vi "Measurement UI.vi"() -> ()   [LabVIEW 2021, in "Line Transient Response with Pin Map UI.lvlib"]
uses:
  Line Transient Response with Pin Map UI.lvlib
  <instrlib>/niScope/Controls/niScope vertical coupling.ctl
  common/UI/controls/UI Scope Parameters.ctl
  common/PMIC Common.lvlib
panel:
  in  "MeasGraphs":T1(tab)
  out "MeasTable":string[][](table)
  out "InputVoltageV/STimeGraph":waveform(dbl)(graph) caption="Load Transient"
  out "OutputVoltageV/STimeGraph":waveform(dbl)(graph) caption="Load Transient"
  in  "Source Voltage v/s Time":string="SOURCE VOLTAGE vs TIME"
  in  "Output Voltage v/s Time":string="LOAD VOLTAGE vs TIME"
  out "ScopeGraph":T2(graph)
  out "waveform pins":string[](array[string])
  in  "enforce realtime":bool[](array[boolean])
  in  "reference position":dbl[](array[numeric]) caption="MIN SAMPLE RATE"
  in  "channel enabled":bool[](array[boolean])
  out "waveform length array":i32[](array[numeric])
  out "waveform dt array":dbl[](array[numeric])
  out "concatenated waveform Y":dbl[](array[numeric])
  out "waveform t0 array":dbl[](array[numeric])
  out "waveform sites":i32[](array[numeric])
  in  "vertical range":dbl[](array[numeric]) caption="VERTICAL RANGE"
  in  "vertical offset":dbl[](array[numeric]) caption="VERTICAL OFFSET"
  in  "probe attenuation":dbl[](array[numeric]) caption="PROBE ATTENUATION"
  in  "vertical coupling":T3[](array[typedef]) caption="VERTICAL COUPLING" items=["AC", "DC", "Ground"]
  in  "input impedance":u32[](array[ring]) caption="INPUT IMPEDANCE" items=["1 mega ohm"=0, "50 ohms"=2]
  in  "max input frequency":dbl[](array[numeric]) caption="MAX INPUT FREQUENCY"
  in  "min sample rate":dbl[](array[numeric]) caption="MIN SAMPLE RATE"
  in  "min record length":i32[](array[numeric]) caption="MIN RECORD LENGTH"
  in  "Pin Names for Scope":string[](array[string]) caption="PIN NAMES"
  out "Overshoot load voltage":dbl
  out "Undershoot load voltage":dbl
  out "Scope amplitudes":dbl[](array[numeric])
  in  "Load transient response":i32(ring)=1042 items=["Slow"=1041, "Normal"=1038, "Fast"=1039, "Custom"=1042]
  out "dt":dbl
  out "Load voltages":dbl[](array[numeric])
  out "Source voltages":dbl[](array[numeric])
  in  "Source transient response":i32(ring)=1042 items=["Slow"=1041, "Normal"=1038, "Fast"=1039, "Custom"=1042]
  in  "Open Scope Dialog":bool
  in  "Load pin name":string caption="LOAD PIN NAME"
  in  "Source pin name":string caption="SOURCE PIN NAME"
  in  "Source model":enum16{"NI PXIe-4151", "NI PXIe-4139"}(ring) caption="RESOURCE MODEL"
  in  "Scope configuration":string="Scope configuration"
  in  "Source voltage delay t2":dbl=0.005 caption="DELAY T2" format="%#_6ps"
  in  "Source voltage delay t1":dbl=0.005 caption="DELAY T1" format="%#_6ps"
  in  "Source voltatge pulse duration":dbl=0.005 caption="PULSE DURATION" format="%#_6ps"
  in  "Source voltage rising slew rate":dbl=50000.0 caption="VOLTAGE RISING SLEW RATE" format="%#_6pV/s"
  in  "Source voltage falling slew rate":dbl=50000.0 caption="VOLTAGE FALLING SLEW RATE" format="%#_6pV/s"
  in  "Source maximum power":dbl=300.0 caption="MAXIMUM POWER" format="%#_6pW"
  in  "Source current limit":dbl=0.25 caption="CURRENT LIMIT" format="%#_6pA"
  in  "Load configuration":string="Load configuration"
  in  "Source configuration":string="Source configuration"
  in  "Source voltage set point 2":dbl=20.0 caption="VOLTAGE SET POINT 2" format="%#_6pV"
  in  "Source voltage set point 1":dbl=7.0 caption="VOLTAGE SET POINT 1" format="%#_6pV"
  in  "Source voltage pole-zero ratio":dbl=2.0 caption="POLE-ZERO RATIO"
  in  "Source voltage gain bandwidth":dbl=2000.0 caption="GAIN BANDWIDTH" format="%#_6pHz"
  in  "Source voltage compensation frequency":dbl=3530.0 caption="COMP. FREQUENCY" format="%#_6pHz"
  in  "Source fast":bool
  in  "Source normal":bool
  in  "Source slow":bool
  in  "Source SourceAdapt":string="Voltage SourceAdapt Parameters"
  in  "Load voltage limit range":dbl=4.0 caption="VOLTAGE LIMIT RANGE" format="%#_6pV"
  in  "Load current level range":dbl=4.0 caption="CURRENT LEVEL RANGE" format="%#_6pA"
  in  "Load current pole-zero ratio":dbl=0.3 caption="POLE-ZERO RATIO"
  in  "Load current gain bandwidth":dbl=14000.0 caption="GAIN BANDWIDTH" format="%#_6pHz"
  in  "Load current compensation frequency":dbl=180000.0 caption="COMP. FREQUENCY" format="%#_6pHz"
  in  "Source sample rate":dbl=1800000.0 caption="SAMPLE RATE" format="%#_6pS/s"
  in  "Load current level":dbl=0.03 caption="CURRENT LEVEL" format="%#_6pA"
  in  "Load fast":bool
  in  "Load normal":bool
  in  "Load slow":bool
  in  "Load SourceAdapt":string="Current SourceAdapt Parameters"
  in  "DUT setup time":dbl=1.0 caption="DUT SETUP TIME" format="%#_6ps"
  in  "Measurement settings":string="Measurement settings"
  in  "Nominal output voltage":dbl=3.3 caption="NOMINAL O/P VOLTAGE" format="%#_6pV"
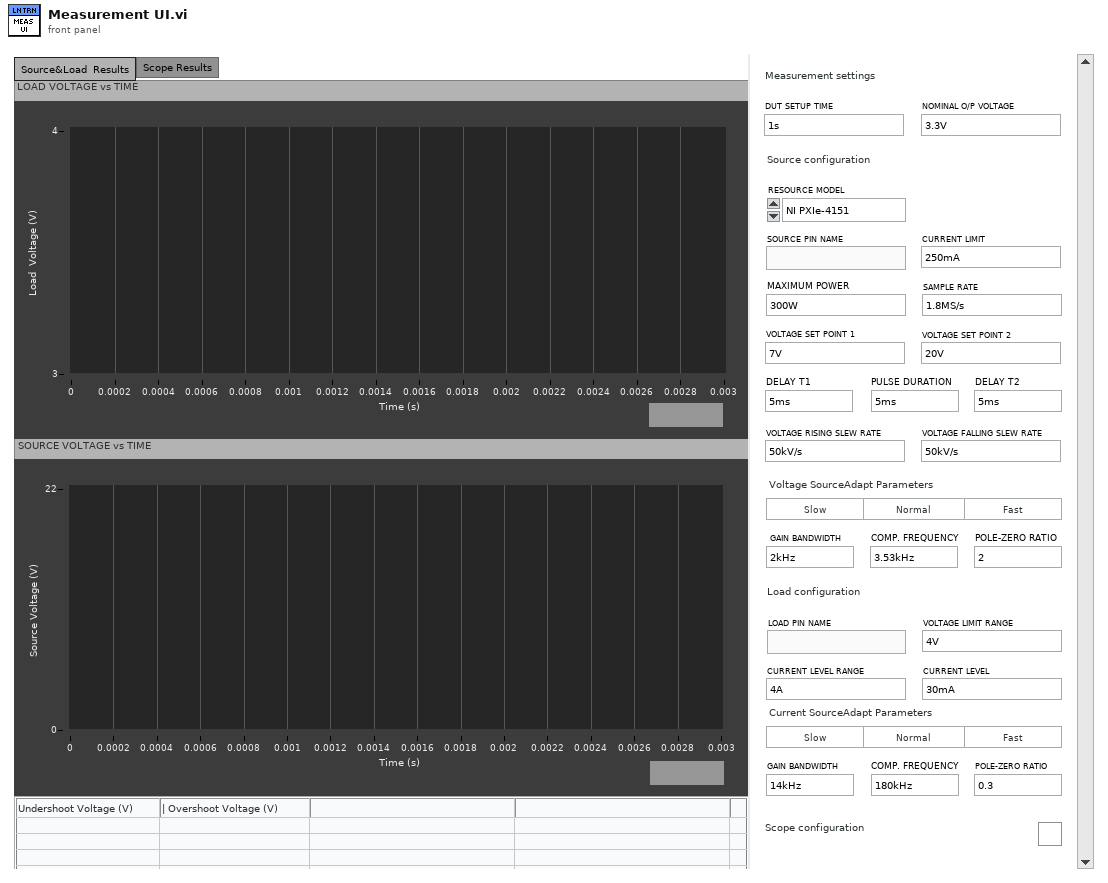
[diagram p1: front panel]
types:
  T1 = enum32{"Source&Load  Results", "Scope Results", "Hidden Controls"}
  T2 = cluster{"Load currents":dbl[], "Efficiency":dbl[]}[]
  T3 = typedef "niScope vertical coupling.ctl" = i32
  T4 = typedef "PMIC Common.lvlib/UI Scope Parameters.ctl" = cluster{"Pin name":string, "Vertical range":dbl, "Vertical offset":dbl, "Probe attenuation":dbl, "Vertical coupling":i32, "Channel enabled":bool, "Input impedance":u32, "Max input frequency":dbl, "Min sample rate":dbl, "Reference position":dbl, "Min record length":i32, "Enforce realtime":bool}
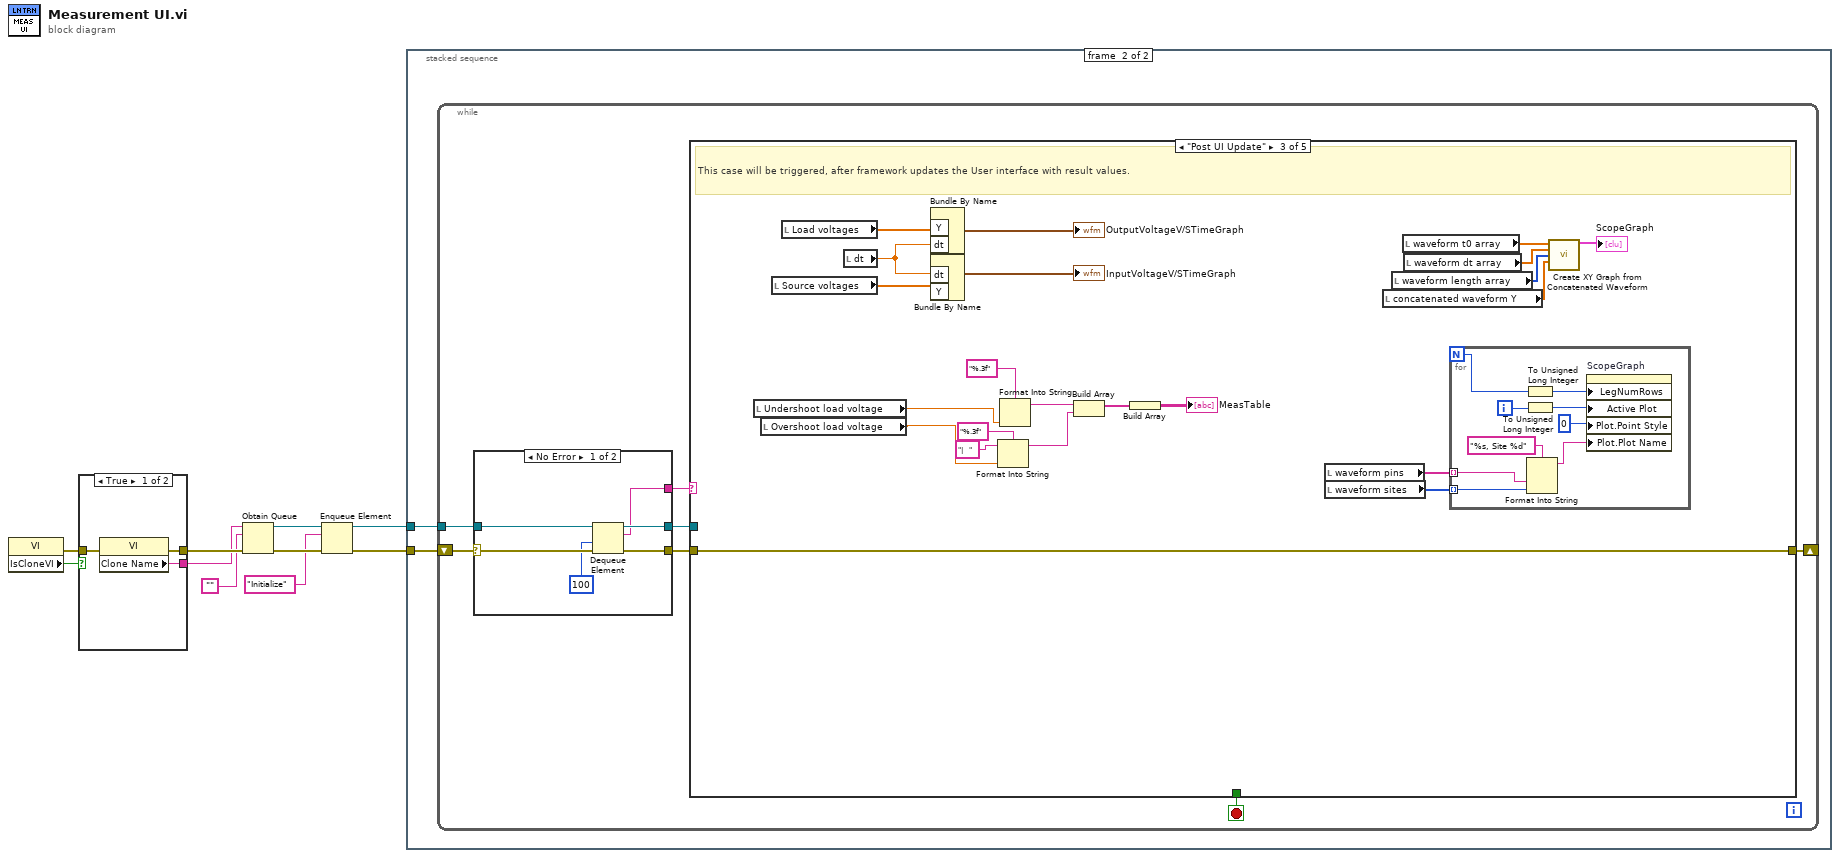
[diagram p0: block diagram]
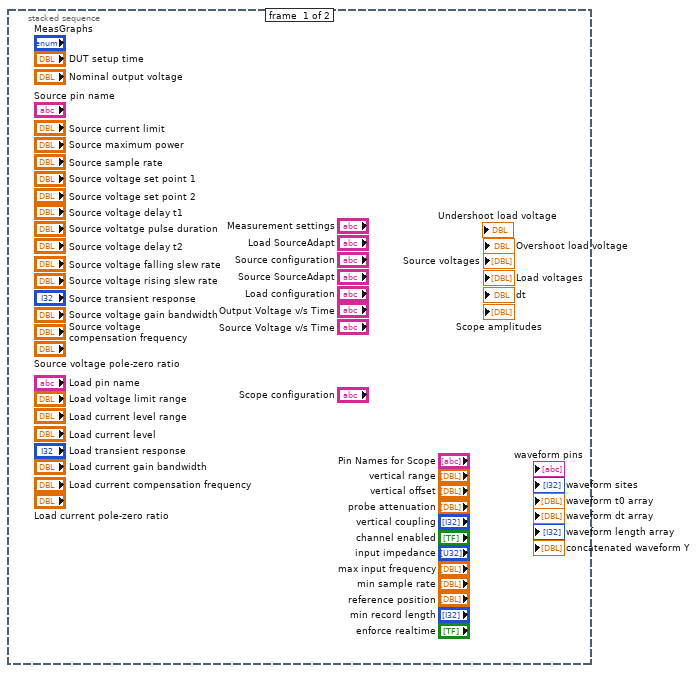
[diagram p2: hidden frame]
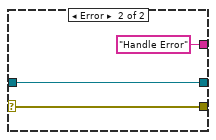
[diagram p3: hidden frame]
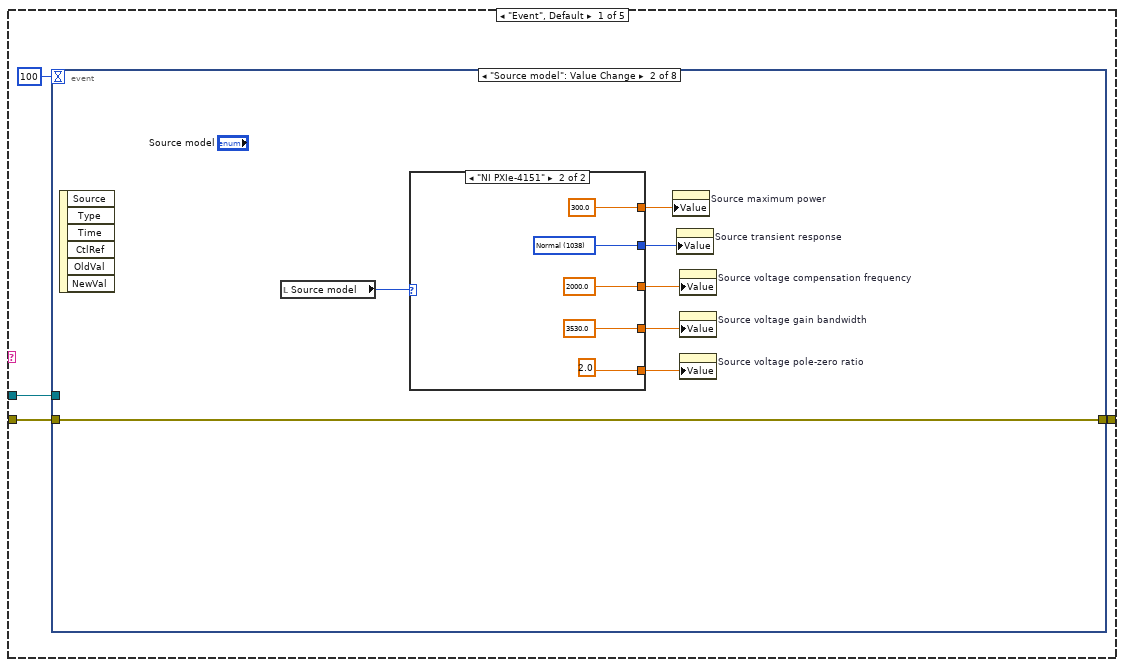
[diagram p4: hidden frame]
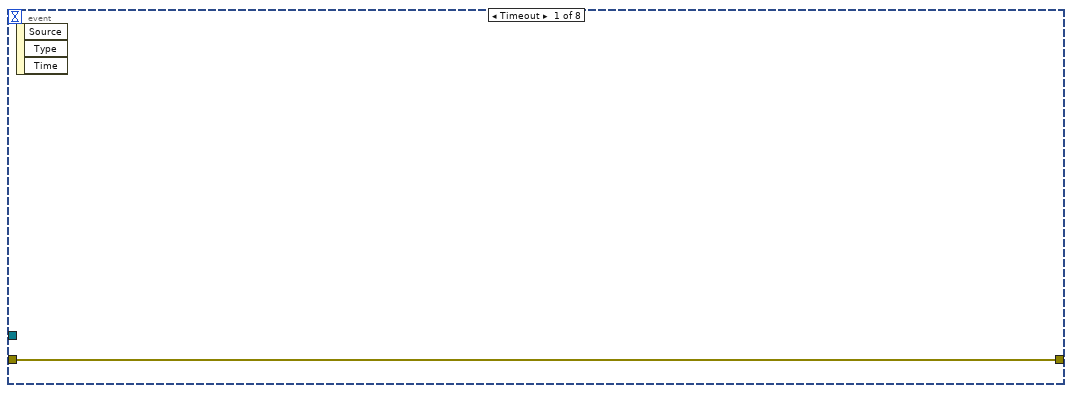
[diagram p5: hidden frame]
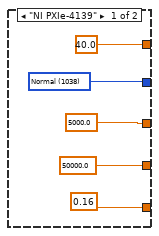
[diagram p6: hidden frame]
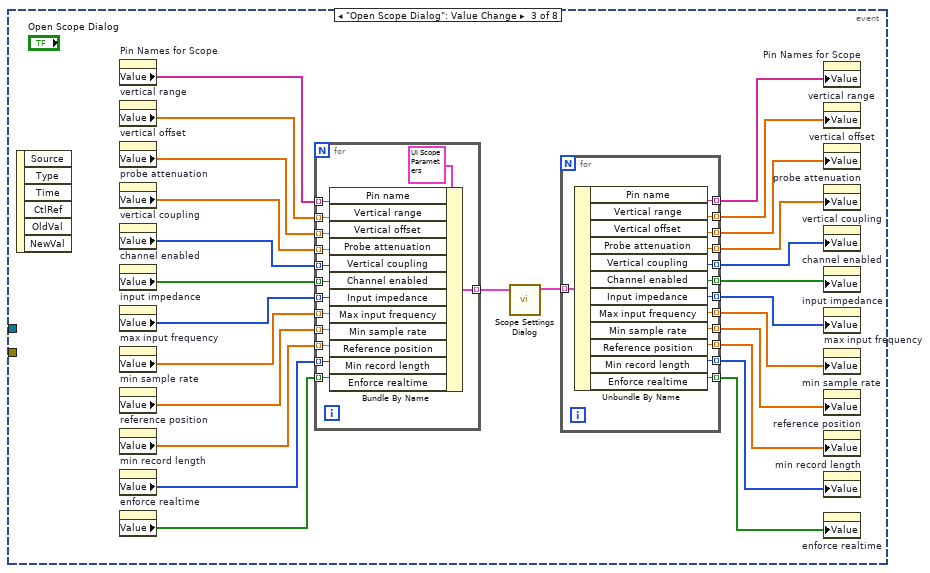
[diagram p7: hidden frame]
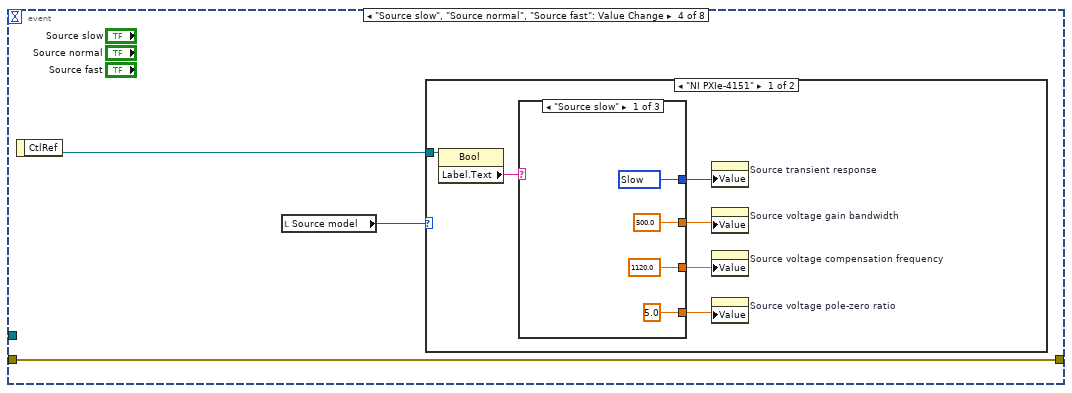
[diagram p8: hidden frame]
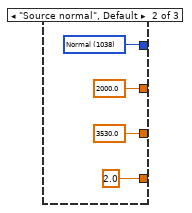
[diagram p9: hidden frame]
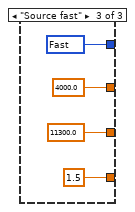
[diagram p10: hidden frame]
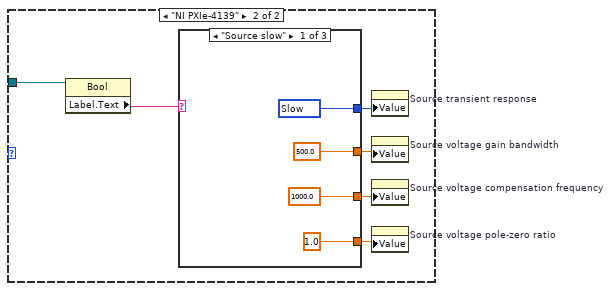
[diagram p11: hidden frame]
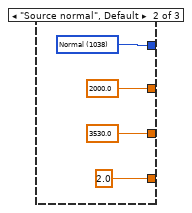
[diagram p12: hidden frame]
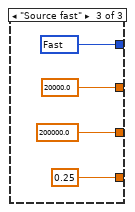
[diagram p13: hidden frame]
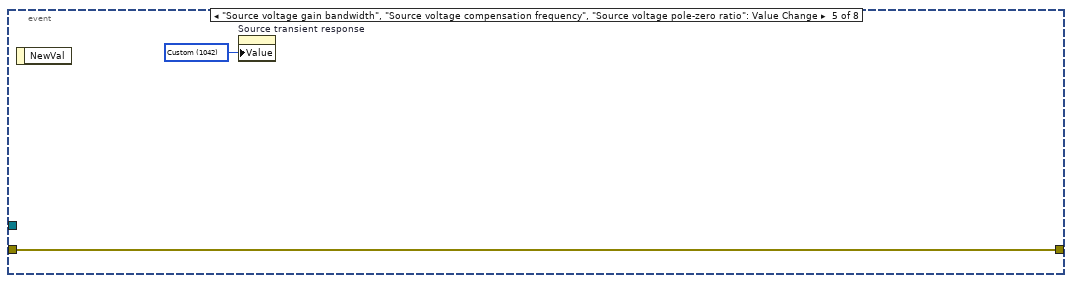
[diagram p14: hidden frame]
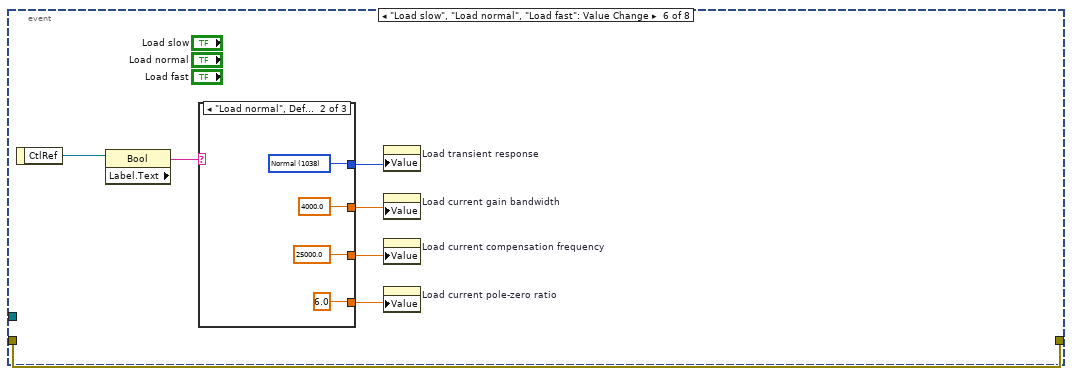
[diagram p15: hidden frame]
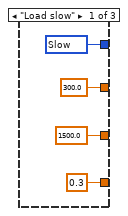
[diagram p16: hidden frame]
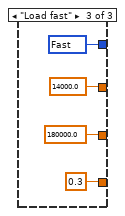
[diagram p17: hidden frame]
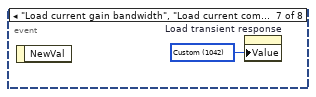
[diagram p18: hidden frame]
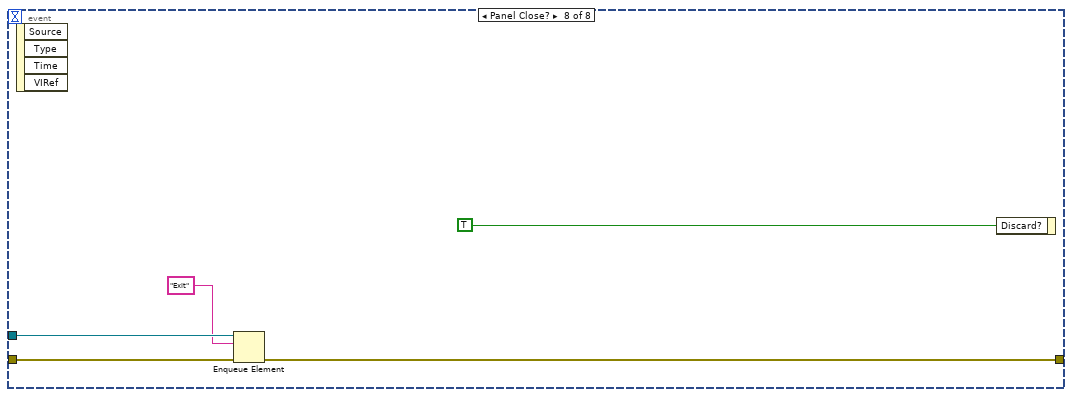
[diagram p19: hidden frame]
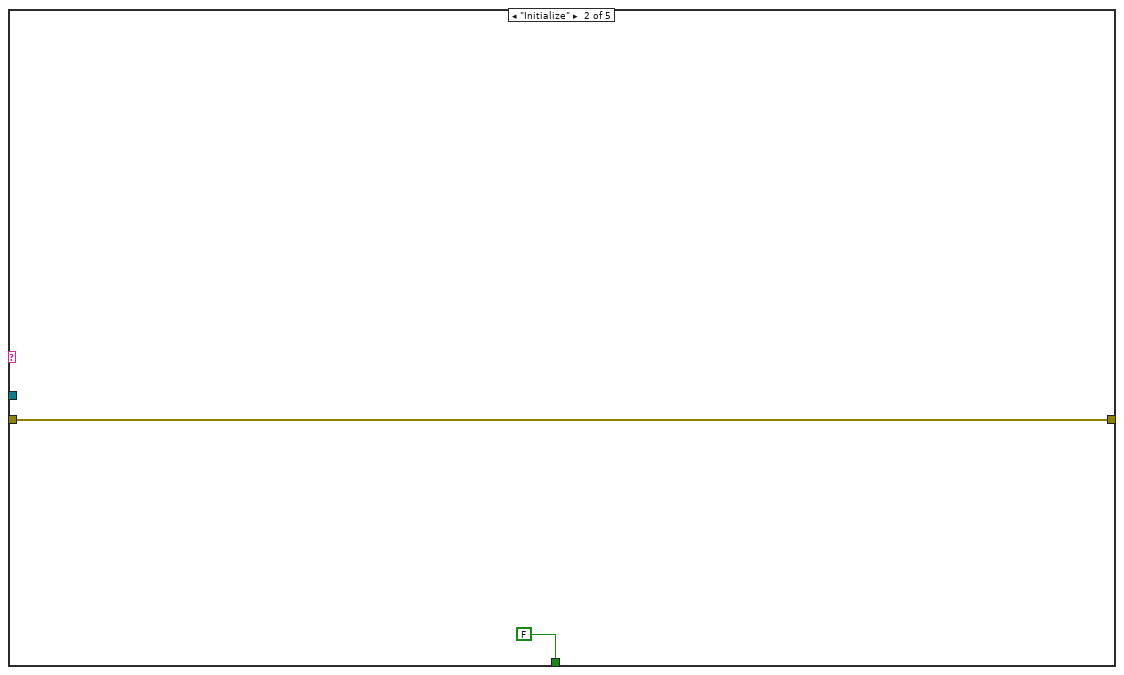
[diagram p20: hidden frame]
diagram:
  n1 = property class="VI"() -> (error out=w1:errorcluster, "IsCloneVI"=w2:bool)  [unwired: 2 in, 1 out]
  n2 = case shown="True" w2 {
    tunnel: [w13 w16] -> w10
    tunnel: [w12 w15] -> w9
    tunnel: w1 -> [w11 w14]
    frame True {
      n3 = property class="VI"(error in=w11) -> (error out=w13:errorcluster, "Clone Name"=w12:string)  [unwired: 1 in, 1 out]
    }
    frame False {
      n4 = property class="VI"(error in=w14) -> (error out=w16:errorcluster, "Name"=w15:string)  [unwired: 1 in, 1 out]
    }
  }
  n5 = Obtain Queue(name (unnamed)=w9, element data type="", error in (no error)=w10) -> (queue out=w6:refnum<queue>, error out=w8:errorcluster)  [unwired: 2 in, 1 out]
  n6 = Enqueue Element(queue=w6, element="Initialize", error in (no error)=w8) -> (queue out=w5:refnum<queue>, error out=w7:errorcluster)  [unwired: 1 in, 1 out]
  n7 = stacked-sequence {
    tunnel: w7 -> [_ w18]
    tunnel: w5 -> [_ w17]
    frame #0 {
    }
    frame #1 {
      n8 = while {
        shift-right: [w20] -> _
        shift-left: w18 -> [w25]
        tunnel: w17 -> [w23]
        stop <- w19 stop-if-true
        n9 = case shown="No Error" w25 {
          selector: w25 -> [w31 w34]
          tunnel: [w30 w34] -> w24
          tunnel: w23 -> [w29 w33]
          tunnel: [w28 w33] -> w22
          tunnel: [w27 "Handle Error"] -> w21
          frame No Error {
            n10 = Dequeue Element(queue=w29, timeout in ms (-1)=100, error in (no error)=w31) -> (queue out=w28:refnum<queue>, element=w27:string, error out=w30:errorcluster)  [unwired: 1 out]
          }
          frame Error {
          }
        }
        n11 = case shown="\"Post UI Update\"" w21 {
          tunnel: w24 -> [w37 w177 w199 w215 w216]
          tunnel: w22 -> [w35 _ _ w213 _]
          tunnel: [w38 w177 w199 w210 w216] -> w20
          tunnel: [_ FALSE _ TRUE _] -> w19
          frame "Event", Default {
            n12 = event shown="[1] \"Source model\": Value Change" {
              selector: _ -> [_ _ _ _ _ _ _ _]
              dyn-events: _ -> [_ _ _ _ _ _ _ _]
              timeout: 100 -> [_ _ _ _ _ _ _ _]
              tunnel: [w39 w46 _ w111 w149 w151 _ w173] -> w38
              tunnel: w37 -> [w39 w46 _ w111 w149 w151 _ w174]
              tunnel: w35 -> [_ _ _ _ _ _ _ w172]
              event Timeout {
                n13 = event-data() -> ()  [unwired: 1 in, 3 out]
              }
              event "Source model": Value Change {
                n14 = event-data() -> ()  [unwired: 1 in, 6 out]
                n15 = local read "Source model"() -> (w40:enum16{"NI PXIe-4151", "NI PXIe-4139"})
                n16 = case shown="\"NI PXIe-4151\"" w40 {
                  tunnel: [40.0 ("Source maximum power") 300.0 ("Source maximum power")] -> w45
                  tunnel: [w50 w55] -> w44
                  tunnel: [5000.0 ("Source maximum power") 2000.0 ("Source maximum power")] -> w43
                  tunnel: [50000.0 ("Source maximum power") 3530.0 ("Source maximum power")] -> w42
                  tunnel: [0.16 ("Source maximum power") 2.0 ("Source maximum power")] -> w41
                  frame "NI PXIe-4139" {
                    w50 = 1038 items=["Slow"=1041, "Normal"=1038, "Fast"=1039, "Custom"=1042] ("Source transient response")
                  }
                  frame "NI PXIe-4151" {
                    w55 = 1038 items=["Slow"=1041, "Normal"=1038, "Fast"=1039, "Custom"=1042] ("Source transient response")
                  }
                }
                n17 = property on="Source maximum power" class="DigNum (strict)"("Value"=w45) -> ()  [unwired: 2 in, 2 out]
                n18 = property on="Source transient response" class="Ring (strict)"("Value"=w44) -> ()  [unwired: 2 in, 2 out]
                n19 = property on="Source voltage compensation frequency" class="DigNum (strict)"("Value"=w43) -> ()  [unwired: 2 in, 2 out]
                n20 = property on="Source voltage gain bandwidth" class="DigNum (strict)"("Value"=w42) -> ()  [unwired: 2 in, 2 out]
                n21 = property on="Source voltage pole-zero ratio" class="DigNum (strict)"("Value"=w41) -> ()  [unwired: 2 in, 2 out]
              }
              event "Open Scope Dialog": Value Change {
                n22 = event-data() -> ()  [unwired: 1 in, 6 out]
                n23 = property on="Pin Names for Scope" class="Arr (strict)"() -> ("Value"=w81:string[])  [unwired: 2 in, 2 out]
                n24 = property on="vertical range" class="Arr (strict)"() -> ("Value"=w80:dbl[])  [unwired: 2 in, 2 out]
                n25 = property on="vertical offset" class="Arr (strict)"() -> ("Value"=w79:dbl[])  [unwired: 2 in, 2 out]
                n26 = property on="probe attenuation" class="Arr (strict)"() -> ("Value"=w78:dbl[])  [unwired: 2 in, 2 out]
                n27 = property on="vertical coupling" class="Arr (strict)"() -> ("Value"=w77:T3[])  [unwired: 2 in, 2 out]
                n28 = property on="channel enabled" class="Arr (strict)"() -> ("Value"=w82:bool[])  [unwired: 2 in, 2 out]
                n29 = property on="input impedance" class="Arr (strict)"() -> ("Value"=w71:u32[])  [unwired: 2 in, 2 out]
                n30 = property on="max input frequency" class="Arr (strict)"() -> ("Value"=w72:dbl[])  [unwired: 2 in, 2 out]
                n31 = property on="min sample rate" class="Arr (strict)"() -> ("Value"=w73:dbl[])  [unwired: 2 in, 2 out]
                n32 = property on="reference position" class="Arr (strict)"() -> ("Value"=w74:dbl[])  [unwired: 2 in, 2 out]
                n33 = property on="min record length" class="Arr (strict)"() -> ("Value"=w75:i32[])  [unwired: 2 in, 2 out]
                n34 = property on="enforce realtime" class="Arr (strict)"() -> ("Value"=w76:bool[])  [unwired: 2 in, 2 out]
                n35 = for {
                  tunnel: w82 -> [w108] mode=indexing
                  tunnel: w81 -> [w107] mode=indexing
                  tunnel: w80 -> [w106] mode=indexing
                  tunnel: w79 -> [w105] mode=indexing
                  tunnel: w78 -> [w104] mode=indexing
                  tunnel: w77 -> [w103] mode=indexing
                  tunnel: w76 -> [w102] mode=indexing
                  tunnel: w75 -> [w101] mode=indexing
                  tunnel: w74 -> [w100] mode=indexing
                  tunnel: w73 -> [w99] mode=indexing
                  tunnel: w72 -> [w98] mode=indexing
                  tunnel: w71 -> [w97] mode=indexing
                  tunnel: [w96] -> w70 mode=indexing
                  n36 = Bundle By Name(cluster=T4 {"Pin name"="", "Vertical range"=10.0, "Vertical offset"=0.0, "Probe attenuation"=1.0, "Vertical coupling"=1, "Channel enabled"=TRUE, "Input impedance"=0, "Max input frequency"=0.0, "Min sample rate"=20000000.0, "Reference position"=50.0, "Min record length"=1000, "Enforce realtime"=TRUE} ("Scope Parameters"), "Pin name"=w107, "Vertical range"=w106, "Vertical offset"=w105, "Probe attenuation"=w104, "Vertical coupling"=w103, "Channel enabled"=w108, "Input impedance"=w97, "Max input frequency"=w98, "Min sample rate"=w99, "Reference position"=w100, "Min record length"=w101, "Enforce realtime"=w102) -> (w96:T4)
                }
                n37 = call "Scope Settings Dialog.vi"("Scope Parameters"=w70) -> ("Scope Parameters out"=w69:T4[])  [unwired: 10 in]
                n38 = for {
                  tunnel: w69 -> [w95] mode=indexing
                  tunnel: [w94] -> w68 mode=indexing
                  tunnel: [w93] -> w67 mode=indexing
                  tunnel: [w92] -> w66 mode=indexing
                  tunnel: [w91] -> w65 mode=indexing
                  tunnel: [w90] -> w64 mode=indexing
                  tunnel: [w89] -> w63 mode=indexing
                  tunnel: [w88] -> w62 mode=indexing
                  tunnel: [w87] -> w61 mode=indexing
                  tunnel: [w86] -> w60 mode=indexing
                  tunnel: [w85] -> w59 mode=indexing
                  tunnel: [w84] -> w58 mode=indexing
                  tunnel: [w83] -> w57 mode=indexing
                  n39 = Unbundle By Name(w95) -> ("Pin name"=w89:string, "Vertical range"=w90:dbl, "Vertical offset"=w91:dbl, "Probe attenuation"=w92:dbl, "Vertical coupling"=w93:i32, "Channel enabled"=w94:bool, "Input impedance"=w88:u32, "Max input frequency"=w87:dbl, "Min sample rate"=w86:dbl, "Reference position"=w85:dbl, "Min record length"=w84:i32, "Enforce realtime"=w83:bool)
                }
                n40 = property on="Pin Names for Scope" class="Arr (strict)"("Value"=w63) -> ()  [unwired: 2 in, 2 out]
                n41 = property on="vertical range" class="Arr (strict)"("Value"=w64) -> ()  [unwired: 2 in, 2 out]
                n42 = property on="vertical offset" class="Arr (strict)"("Value"=w65) -> ()  [unwired: 2 in, 2 out]
                n43 = property on="probe attenuation" class="Arr (strict)"("Value"=w66) -> ()  [unwired: 2 in, 2 out]
                n44 = property on="vertical coupling" class="Arr (strict)"("Value"=w67) -> ()  [unwired: 2 in, 2 out]
                n45 = property on="channel enabled" class="Arr (strict)"("Value"=w68) -> ()  [unwired: 2 in, 2 out]
                n46 = property on="input impedance" class="Arr (strict)"("Value"=w62) -> ()  [unwired: 2 in, 2 out]
                n47 = property on="max input frequency" class="Arr (strict)"("Value"=w61) -> ()  [unwired: 2 in, 2 out]
                n48 = property on="min sample rate" class="Arr (strict)"("Value"=w60) -> ()  [unwired: 2 in, 2 out]
                n49 = property on="reference position" class="Arr (strict)"("Value"=w59) -> ()  [unwired: 2 in, 2 out]
                n50 = property on="min record length" class="Arr (strict)"("Value"=w58) -> ()  [unwired: 2 in, 2 out]
                n51 = property on="enforce realtime" class="Arr (strict)"("Value"=w57) -> ()  [unwired: 2 in, 2 out]
              }
              event "Source slow", "Source normal", "Source fast": Value Change {
                n52 = event-data() -> ("CtlRef"=w112:refnum<vi>)  [unwired: 1 in]
                n53 = local read "Source model"() -> (w110:enum16{"NI PXIe-4151", "NI PXIe-4139"})
                n54 = case shown="\"NI PXIe-4151\"" w110 {
                  tunnel: w112 -> [w113 w131]
                  frame "NI PXIe-4151" {
                    n55 = property class="Bool"(reference=w113) -> ("Label.Text"=w118:string)  [unwired: 1 in, 2 out]
                    n56 = case shown="\"Source slow\"" w118 {
                      tunnel: [w122 w126 w130] -> w117
                      tunnel: [500.0 ("Source voltage gain bandwidth") 2000.0 ("Source voltage gain bandwidth") 4000.0 ("Source voltage gain bandwidth")] -> w116
                      tunnel: [1120.0 ("Source voltage compensation frequency") 3530.0 ("Source voltage compensation frequency") 11300.0 ("Source voltage compensation frequency")] -> w115
                      tunnel: [5.0 ("Source voltage pole-zero ratio") 2.0 ("Source voltage pole-zero ratio") 1.5 ("Source voltage pole-zero ratio")] -> w114
                      frame "Source slow" {
                        w122 = 1041 items=["Slow"=1041, "Normal"=1038, "Fast"=1039, "Custom"=1042] ("Source transient response")
                      }
                      frame "Source normal", Default {
                        w126 = 1038 items=["Slow"=1041, "Normal"=1038, "Fast"=1039, "Custom"=1042] ("Source transient response")
                      }
                      frame "Source fast" {
                        w130 = 1039 items=["Slow"=1041, "Normal"=1038, "Fast"=1039, "Custom"=1042] ("Source transient response")
                      }
                    }
                    n57 = property on="Source transient response" class="Ring (strict)"("Value"=w117) -> ()  [unwired: 2 in, 2 out]
                    n58 = property on="Source voltage gain bandwidth" class="DigNum (strict)"("Value"=w116) -> ()  [unwired: 2 in, 2 out]
                    n59 = property on="Source voltage compensation frequency" class="DigNum (strict)"("Value"=w115) -> ()  [unwired: 2 in, 2 out]
                    n60 = property on="Source voltage pole-zero ratio" class="DigNum (strict)"("Value"=w114) -> ()  [unwired: 2 in, 2 out]
                  }
                  frame "NI PXIe-4139" {
                    n61 = property class="Bool"(reference=w131) -> ("Label.Text"=w136:string)  [unwired: 1 in, 2 out]
                    n62 = case shown="\"Source slow\"" w136 {
                      tunnel: [w140 w144 w148] -> w135
                      tunnel: [500.0 ("Source voltage gain bandwidth") 2000.0 ("Source voltage gain bandwidth") 20000.0 ("Source voltage gain bandwidth")] -> w134
                      tunnel: [1000.0 ("Source voltage compensation frequency") 3530.0 ("Source voltage compensation frequency") 200000.0 ("Source voltage compensation frequency")] -> w133
                      tunnel: [1.0 ("Source voltage pole-zero ratio") 2.0 ("Source voltage pole-zero ratio") 0.25 ("Source voltage pole-zero ratio")] -> w132
                      frame "Source slow" {
                        w140 = 1041 items=["Slow"=1041, "Normal"=1038, "Fast"=1039, "Custom"=1042] ("Source transient response")
                      }
                      frame "Source normal", Default {
                        w144 = 1038 items=["Slow"=1041, "Normal"=1038, "Fast"=1039, "Custom"=1042] ("Source transient response")
                      }
                      frame "Source fast" {
                        w148 = 1039 items=["Slow"=1041, "Normal"=1038, "Fast"=1039, "Custom"=1042] ("Source transient response")
                      }
                    }
                    n63 = property on="Source transient response" class="Ring (strict)"("Value"=w135) -> ()  [unwired: 2 in, 2 out]
                    n64 = property on="Source voltage gain bandwidth" class="DigNum (strict)"("Value"=w134) -> ()  [unwired: 2 in, 2 out]
                    n65 = property on="Source voltage compensation frequency" class="DigNum (strict)"("Value"=w133) -> ()  [unwired: 2 in, 2 out]
                    n66 = property on="Source voltage pole-zero ratio" class="DigNum (strict)"("Value"=w132) -> ()  [unwired: 2 in, 2 out]
                  }
                }
              }
              event "Source voltage gain bandwidth", "Source voltage compensation frequency", "Source voltage pole-zero ratio": Value Change {
                w150 = 1042 items=["Slow"=1041, "Normal"=1038, "Fast"=1039, "Custom"=1042] ("Source transient response")
                n67 = event-data() -> ()  [unwired: 1 in, 1 out]
                n68 = property on="Source transient response" class="Ring (strict)"("Value"=w150) -> ()  [unwired: 2 in, 2 out]
              }
              event "Load slow", "Load normal", "Load fast": Value Change {
                n69 = event-data() -> ("CtlRef"=w152:refnum<vi>)  [unwired: 1 in]
                n70 = property class="Bool"(reference=w152) -> ("Label.Text"=w157:string)  [unwired: 1 in, 2 out]
                n71 = case shown="\"Load normal\", Default" w157 {
                  tunnel: [w161 w165 w169] -> w156
                  tunnel: [300.0 ("Load current gain bandwidth") 4000.0 ("Load current gain bandwidth") 14000.0 ("Load current gain bandwidth")] -> w155
                  tunnel: [1500.0 ("Load current compensation frequency") 25000.0 ("Load current compensation frequency") 180000.0 ("Load current compensation frequency")] -> w154
                  tunnel: [0.3 ("Load current pole-zero ratio") 6.0 ("Load current pole-zero ratio") 0.3 ("Load current pole-zero ratio")] -> w153
                  frame "Load slow" {
                    w161 = 1041 items=["Slow"=1041, "Normal"=1038, "Fast"=1039, "Custom"=1042] ("Source transient response")
                  }
                  frame "Load normal", Default {
                    w165 = 1038 items=["Slow"=1041, "Normal"=1038, "Fast"=1039, "Custom"=1042] ("Source transient response")
                  }
                  frame "Load fast" {
                    w169 = 1039 items=["Slow"=1041, "Normal"=1038, "Fast"=1039, "Custom"=1042] ("Source transient response")
                  }
                }
                n72 = property on="Load transient response" class="Ring (strict)"("Value"=w156) -> ()  [unwired: 2 in, 2 out]
                n73 = property on="Load current gain bandwidth" class="DigNum (strict)"("Value"=w155) -> ()  [unwired: 2 in, 2 out]
                n74 = property on="Load current compensation frequency" class="DigNum (strict)"("Value"=w154) -> ()  [unwired: 2 in, 2 out]
                n75 = property on="Load current pole-zero ratio" class="DigNum (strict)"("Value"=w153) -> ()  [unwired: 2 in, 2 out]
              }
              event "Load current gain bandwidth", "Load current compensation frequency", "Load current pole-zero ratio": Value Change {
                w170 = 1042 items=["Slow"=1041, "Normal"=1038, "Fast"=1039, "Custom"=1042] ("Load transient response")
                n76 = event-data() -> ()  [unwired: 1 in, 1 out]
                n77 = property on="Load transient response" class="Ring (strict)"("Value"=w170) -> ()  [unwired: 2 in, 2 out]
              }
              event Panel Close? {
                n78 = event-data() -> ()  [unwired: 1 in, 4 out]
                n79 = Enqueue Element(queue=w172, element="Exit", error in (no error)=w174) -> (error out=w173:errorcluster)  [unwired: 1 in, 2 out]
                n80 = event-data("Discard?"=TRUE) -> ()  [unwired: 1 in, 1 out]
              }
            }
          }
          frame "Initialize" {
          }
          frame "Post UI Update" {
            # "This case will be triggered, after framework updates the User interface with result values."
            n81 = local read "Undershoot load voltage"() -> (w189:dbl)
            n82 = local read "Overshoot load voltage"() -> (w188:dbl)
            n83 = local read "Source voltages"() -> (w195:dbl[])
            n84 = local read "Load voltages"() -> (w198:dbl[])
            n85 = local read "dt"() -> (w193:dbl)
            n86 = Bundle By Name("Y"=w198, "dt"=w193) -> (→"OutputVoltageV/STimeGraph":waveform(dbl))  [unwired: 1 in]
            n87 = Bundle By Name("dt"=w193, "Y"=w195) -> (→"InputVoltageV/STimeGraph":waveform(dbl))  [unwired: 1 in]
            n88 = Format Into String(format string="%.3f" ("initial string"), initial string="|   ", w188) -> (resulting string=w187:string)  [unwired: 1 in, 1 out]
            n89 = Format Into String(format string="%.3f" ("initial string"), w189) -> (resulting string=w194:string)  [unwired: 2 in, 1 out]
            n90 = Build Array(w194, w187) -> (w186:string[])
            n91 = Build Array(w186) -> (→"MeasTable":string[][])
            n92 = local read "waveform pins"() -> (w184:string[])
            n93 = local read "waveform sites"() -> (w183:i32[])
            n94 = local read "concatenated waveform Y"() -> (w179:dbl[])
            n95 = local read "waveform length array"() -> (w180:i32[])
            n96 = local read "waveform t0 array"() -> (w182:dbl[])
            n97 = local read "waveform dt array"() -> (w181:dbl[])
            n98 = for {
              N -> [w206]
              tunnel: w183 -> [w205] mode=indexing
              tunnel: w184 -> [w204] mode=indexing
              i -> [w207]
              n99 = To Unsigned Long Integer(number=w206) -> (unsigned 32bit integer=w203:u32)
              n100 = To Unsigned Long Integer(number=w207) -> (unsigned 32bit integer=w202:u32)
              n101 = Format Into String(format string="%s, Site %d", w204, w205) -> (resulting string=w200:string)  [unwired: 2 in, 1 out]
              n102 = property on="ScopeGraph" class="XYGraph (strict)"("LegNumRows"=w203, "Active Plot"=w202, "Plot.Point Style"=u8 0, "Plot.Plot Name"=w200) -> ()  [unwired: 2 in, 2 out]
            }
            n103 = call "Create XY Graph from Concatenated Waveform.vi"("waveform t0 array"=w182, "waveform dt array"=w181, "waveform length array"=w180, "concatenated waveform Y"=w179) -> ("XY Graph Array"=→"ScopeGraph":cluster{"time":dbl[], "waveform":dbl[]}[])  [unwired: 11 in]
          }
          frame "Exit" {
            # "This case is triggered to close the User Interface from framework"
            n104 = Flush Queue(queue=w213, error in (no error)=w215) -> (queue out=w212:refnum<queue>, error out=w211:errorcluster)  [unwired: 1 out]
            n105 = Release Queue(queue=w212, force destroy? (F)=TRUE, error in (no error)=w211) -> (error out=w210:errorcluster)  [unwired: 2 out]
          }
          frame "Handle Error" {
          }
        }
      }
    }
  }
